vi "Get Property Data (U64).vi"(8 "error in":errorcluster, 10 "Property Name":string, 11 "Item in":refnum<class "Item.lvclass">) -> (0 "error out":errorcluster, 3 "Property Value":u64)   [LabVIEW 2024, in "Parser.lvlib" / "Property.lvclass"]
uses:
  Property.lvclass
  Item/Item.lvclass
  Controls/Property Type.ctl
  Item/Item.lvclass/Item.ctl
  Property.lvclass/Property.ctl
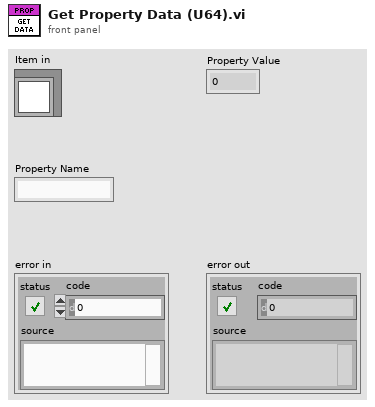
[diagram p1: front panel]
types:
  T1 = typedef "Parser.lvlib/Property.lvclass/Property Type.ctl" = enum16{"Boolean", "Double", "String", "Path", "Dictionary", "DependentFile", "I16", "I32", "I64", "U16", "U32", "U64", "BooleanArray", "DoubleArray", "StringArray", "I16Array", "I32Array", "I64Array", "U16Array", "U32Array", "U64Array", "Variant"}
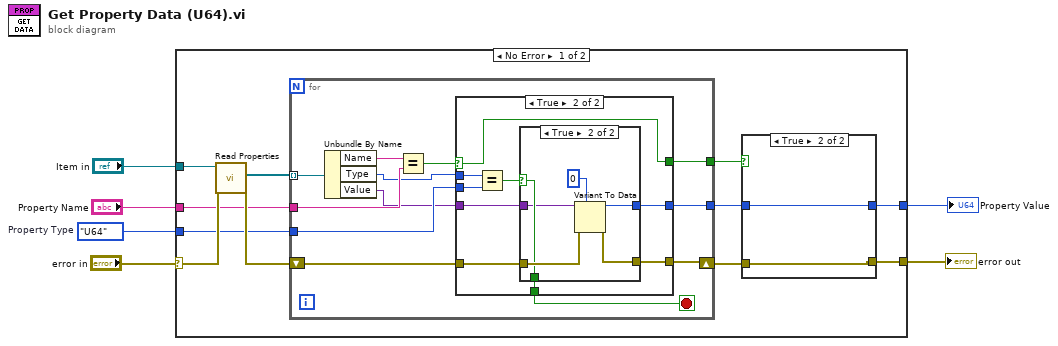
[diagram p0: block diagram]
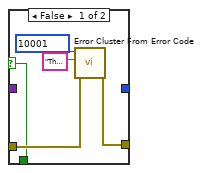
[diagram p3: hidden frame]
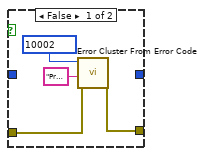
[diagram p4: hidden frame]
diagram:
  w3 = Property_Type."U64"  # Property Type
  n1 = case shown="No Error" "error in" {
    selector: "error in" -> [w14 w58]
    tunnel: [w17 w58] -> w6
    tunnel: "Property Name" -> [w13 _]
    tunnel: w3 -> [w12 _]
    tunnel: "Item in" -> [w8 _]
    tunnel: [w7 _] -> w1
    frame No Error {
      n2 = call "Read Properties.vi"("error in"=w14, "Item in"=w8) -> ("error out"=w16:errorcluster, "Properties"=w9:refnum<class "Property.lvclass">[])  [unwired: 7 in, 1 out]
      n3 = for {
        tunnel: w13 -> [w25]
        tunnel: w12 -> [w22]
        tunnel: [w23] -> w11
        tunnel: [w21] -> w10
        tunnel: w9 -> [w20] mode=indexing
        shift-right: [w28] -> w15
        shift-left: w16 -> [w29]
        stop <- w18 stop-if-true
        n4 = Unbundle By Name(w20) -> ("Name"=w26:string, "Type"=w24:T1, "Value"=w19:variant)
        n5 = Equal?(x=w26, y=w25) -> (x = y?=w27:bool)
        n6 = case shown="True" w27 {
          selector: w27 -> [w30 w33]
          tunnel: [_ w38] -> w21
          tunnel: w19 -> [_ w37]
          tunnel: w22 -> [_ w35]
          tunnel: w24 -> [_ w36]
          tunnel: [w30 w33] -> w23
          tunnel: [w30 w32] -> w18
          tunnel: w29 -> [w31 w40]
          tunnel: [w31 w39] -> w28
          frame False {
          }
          frame True {
            n7 = Equal?(x=w36, y=w35) -> (x = y?=w34:bool)
            n8 = case shown="True" w34 {
              selector: w34 -> [w41 w48]
              tunnel: [_ w49] -> w38
              tunnel: w37 -> [_ w47]
              tunnel: [w41 w48] -> w32
              tunnel: w40 -> [w45 w51]
              tunnel: [w44 w50] -> w39
              frame False {
                n9 = call <vilib>:"Error Cluster From Error Code.vi"("error in (no error)"=w45, "error message (\"\")"="The selected type is incompatible with the chosen property", "error code (0)"=10001) -> ("error out"=w44:errorcluster)  [unwired: 6 in]
              }
              frame True {
                n10 = Variant To Data(error in=w51, type=u64 0, Variant=w47) -> (data=w49:u64, error out=w50:errorcluster)
              }
            }
          }
        }
      }
      n11 = case shown="True" w11 {
        tunnel: w10 -> [_ w56]
        tunnel: [_ w56] -> w7
        tunnel: [w55 w57] -> w17
        tunnel: w15 -> [w54 w57]
        frame False {
          n12 = call <vilib>:"Error Cluster From Error Code.vi"("error in (no error)"=w54, "error message (\"\")"="Property does not exist", "error code (0)"=10002) -> ("error out"=w55:errorcluster)  [unwired: 6 in]
        }
        frame True {
        }
      }
    }
    frame Error {
    }
  }
  "error out" <- w6
  "Property Value" <- w1
